vi "getWIPStatus.vi"(10 "Lotno":string) -> (2 "Status":string, 3 "step":string)   [LabVIEW 2012]
uses:
  <vilib>/addons/database/Auxilliary.llb/DB Tools Cursor Type.ctl
  <vilib>/addons/database/Connection.llb/DB Tools Open Connec (Path).vi
  <vilib>/addons/database/Connection.llb/Conn Execute.vi
  <vilib>/addons/database/Recordset.llb/Rec Fetch Integer Data (R).vi
  <vilib>/addons/database/Recordset.llb/Rec Destroy - Connection.vi
  <vilib>/addons/database/Recordset.llb/Rec Fetch Recordset Data (R).vi
  <vilib>/addons/database/_DB Variant To Data/Database Variant To Data.xnode
  <vilib>/addons/database/NI_Database_API.lvlib
panel:
  out "CustomerID":string
  out "BATCHQTY":i32
  out "SSEBATCH":string
  out "location":string
  out "lotno":string
  out "Package":string
  out "data":i32
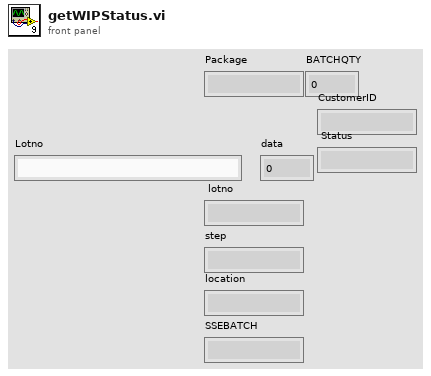
[diagram p1: front panel]
types:
  T1 = typedef "NI_Database_API.lvlib/DB Tools Cursor Type.ctl" = enum16{"forward-only", "keyset", "dynamic", "static"}
  T2 = typedef "NI_Database_API.lvlib/Conn ObjectReference.ctl" = refnum<k1>
  T3 = typedef "NI_Database_API.lvlib/Rec ObjectReference.ctl" = refnum<k1>
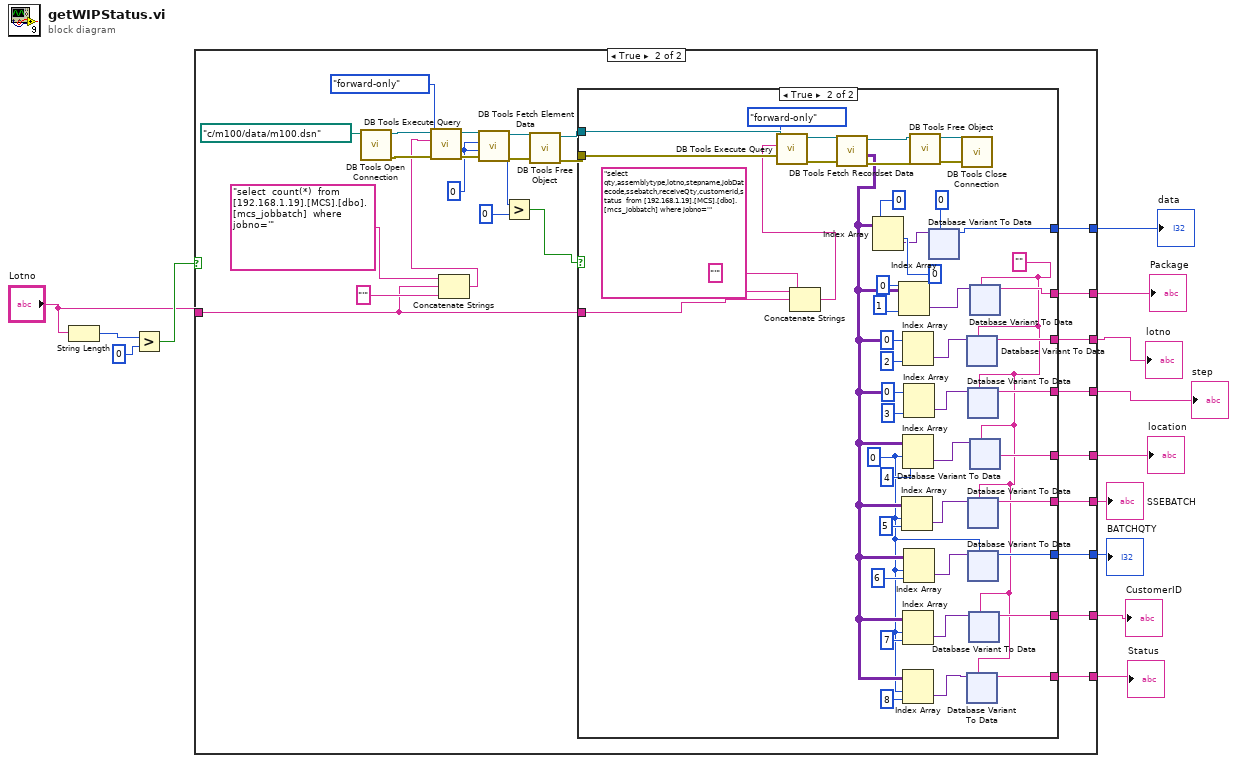
[diagram p0: block diagram]
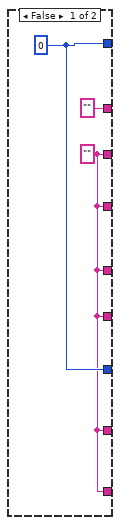
[diagram p2: hidden frame]
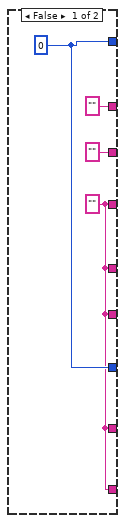
[diagram p3: hidden frame]
diagram:
  n1 = String Length(string="Lotno") -> (length=w13:i32)
  n2 = Greater?(x=w13, y=0) -> (0:w11:bool)
  n3 = case shown="True" w11 {
    tunnel: "Lotno" -> [_ w33]
    tunnel: [w14 w43] -> w9
    tunnel: ["" ("data") w42] -> w8
    tunnel: [w15 w41] -> w7
    tunnel: [w14 w40] -> w6
    tunnel: [w14 w22] -> w5
    tunnel: [w14 w21] -> w4
    tunnel: [w15 w20] -> w3
    tunnel: [w14 w19] -> w2
    tunnel: [w14 w18] -> w1
    frame False {
      w14 = "" ("data")
      w15 = 0 ("data")
    }
    frame True {
      w26 = 0
      n4 = call-poly <vilib>:"DB Tools Open Connection.vi"("connection information"=path "c:/m100/data/m100.dsn") -> ("error out"=w36:errorcluster, "connection reference"=w37:T2)  [unwired: 7 in]
      n5 = Concatenate Strings("select  count(*)  from [192.168.1.19].[MCS].[dbo].[mcs_jobbatch]  where jobno='" ("string"), w33, "'" ("string")) -> (w31:string)
      n6 = call-poly <vilib>:"DB Tools Execute Query.vi"("error in (no error)"=w36, "cursor type"=DB_Tools_Cursor_Type."forward-only", "SQL query"=w31, "connection reference"=w37) -> ("error out"=w30:errorcluster, "recordset reference"=w29:T3)  [unwired: 4 in]
      n7 = call-poly <vilib>:"DB Tools Fetch Element Data.vi"("error in (no error)"=w30, "type"=w26, "column index"=w26, "recordset reference"=w29) -> ("error out"=w27:errorcluster, "data"=w25:i32, "recordset reference out"=w28:T3)  [unwired: 3 in]
      n8 = Greater?(x=w25, y=0) -> (0:w23:bool)
      n9 = call-poly <vilib>:"DB Tools Free Object.vi"("error in (no error)"=w27, "recordset reference"=w28) -> ("error out"=w38:errorcluster, "connection reference"=w39:T2)  [unwired: 8 in]
      n10 = case shown="True" w23 {
        tunnel: w39 -> [_ w93]
        tunnel: w38 -> [_ w90]
        tunnel: w33 -> [_ w73]
        tunnel: ["" ("data") w72] -> w43
        tunnel: ["" ("data") w71] -> w42
        tunnel: [w45 w70] -> w41
        tunnel: [w44 w66] -> w40
        tunnel: [w44 w63] -> w22
        tunnel: [w44 w58] -> w21
        tunnel: [w45 w57] -> w20
        tunnel: [w44 w54] -> w19
        tunnel: [w44 w48] -> w18
        frame False {
          w44 = "" ("data")
          w45 = 0 ("data")
        }
        frame True {
          w52 = 0 ("index (row)")
          w49 = ""
          n11 = Concatenate Strings("select qty,assemblytype,lotno,stepname,jobDatecode,ssebatch,receiveQty,customerid,status  from [192.168.1.19].[MCS].[dbo].[mcs_jobbatch] where jobno='" ("string"), w73, "'" ("string")) -> (w84:string)
          n12 = call-poly <vilib>:"DB Tools Execute Query.vi"("error in (no error)"=w90, "cursor type"=DB_Tools_Cursor_Type."forward-only", "SQL query"=w84, "connection reference"=w93) -> ("error out"=w89:errorcluster, "recordset reference"=w92:T3)  [unwired: 4 in]
          n13 = call-poly <vilib>:"DB Tools Fetch Recordset Data.vi"("error in (no error)"=w89, "recordset reference"=w92) -> ("error out"=w88:errorcluster, "recordset data"=w53:variant[][], "recordset reference out"=w91:T3)  [unwired: 3 in]
          n14 = Index Array(array=w53, index (row)=0, index (col)=0 ("disabled index (col)")) -> (element=w81:variant)
          n15 = Index Array(array=w53, index (row)=0 ("disabled index (row)"), index (col)=1 ("disabled index (col)")) -> (element=w77:variant)
          n16 = Index Array(array=w53, index (row)=w52, index (col)=5 ("disabled index (col)")) -> (element=w60:variant)
          n17 = Index Array(array=w53, index (row)=0 ("disabled index (row)"), index (col)=2 ("disabled index (col)")) -> (element=w76:variant)
          n18 = Index Array(array=w53, index (row)=w52, index (col)=4 ("disabled index (col)")) -> (element=w64:variant)
          n19 = Index Array(array=w53, index (row)=w52, index (col)=7 ("disabled index (col)")) -> (element=w55:variant)
          n20 = Index Array(array=w53, index (row)=w52, index (col)=8 ("disabled index (col)")) -> (element=w50:variant)
          n21 = Index Array(array=w53, index (row)=0 ("disabled index (row)"), index (col)=3 ("disabled index (col)")) -> (element=w67:variant)
          n22 = Index Array(array=w53, index (row)=w52, index (col)=6 ("disabled index (col)")) -> (element=w59:variant)
          n23 = call-poly <vilib>:"DB Tools Free Object.vi"("error in (no error)"=w88, "recordset reference"=w91) -> ("error out"=w95:errorcluster, "connection reference"=w94:T2)  [unwired: 8 in]
          n24 = xnode "Database Variant To Data"("database variant"=w81, "type"=0) -> ("data"=w70:i32)  [unwired: 1 in, 1 out]
          n25 = call <vilib>:"DB Tools Close Connection.vi"("error in (no error)"=w95, "connection reference"=w94) -> ()  [unwired: 5 in, 1 out]
          n26 = xnode "Database Variant To Data"("database variant"=w76, "type"=w49) -> ("data"=w72:string)  [unwired: 1 in, 1 out]
          n27 = xnode "Database Variant To Data"("database variant"=w50, "type"=w49) -> ("data"=w48:string)  [unwired: 1 in, 1 out]
          n28 = xnode "Database Variant To Data"("database variant"=w67, "type"=w49) -> ("data"=w66:string)  [unwired: 1 in, 1 out]
          n29 = xnode "Database Variant To Data"("database variant"=w60, "type"=w49) -> ("data"=w58:string)  [unwired: 1 in, 1 out]
          n30 = xnode "Database Variant To Data"("database variant"=w59, "type"=w52) -> ("data"=w57:i32)  [unwired: 1 in, 1 out]
          n31 = xnode "Database Variant To Data"("database variant"=w55, "type"=w49) -> ("data"=w54:string)  [unwired: 1 in, 1 out]
          n32 = xnode "Database Variant To Data"("database variant"=w77, "type"=w49) -> ("data"=w71:string)  [unwired: 1 in, 1 out]
          n33 = xnode "Database Variant To Data"("database variant"=w64, "type"=w49) -> ("data"=w63:string)  [unwired: 1 in, 1 out]
        }
      }
    }
  }
  "data" <- w7
  "Package" <- w8
  "lotno" <- w9
  "step" <- w6
  "location" <- w5
  "SSEBATCH" <- w4
  "BATCHQTY" <- w3
  "CustomerID" <- w2
  "Status" <- w1
